vi "LVClasse_Phase Read SurfaceFloatWithPupil.vi"(8 "error in (no error)":errorcluster, 11 "Phase in":refnum<class "Phase.lvclass">) -> (0 "error out":errorcluster, 2 "SurfaceFloatWithPupil":i32, 3 "Phase out":refnum<class "Phase.lvclass">)   [LabVIEW 2020, in "Phase.lvclass"]
uses:
  Phase.lvclass
  Phase.lvclass/Phase.ctl
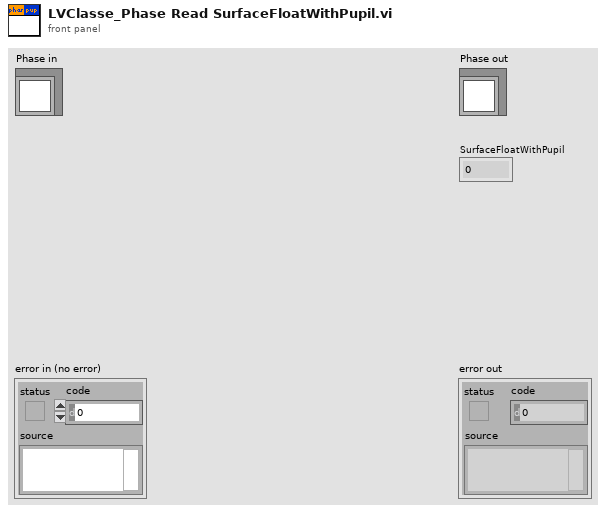
[diagram p1: front panel]
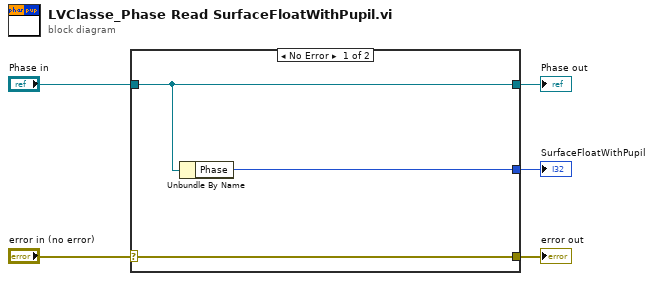
[diagram p0: block diagram]
diagram:
  n1 = case shown="No Error" "error in (no error)" {
    selector: "error in (no error)" -> [w8 w9]
    tunnel: [w8 w9] -> w4
    tunnel: [w7 w10] -> w2
    tunnel: "Phase in" -> [w7 w10]
    tunnel: [w6 _] -> w1
    frame No Error {
      n2 = Unbundle By Name(w7) -> ("Phase"=w6:i32)
    }
    frame Error {
    }
  }
  "error out" <- w4
  "Phase out" <- w2
  "SurfaceFloatWithPupil" <- w1
